vi "timeTest.vi"() -> ()   [LabVIEW 2019]
panel:
  out "czas":u32
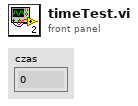
[diagram p1: front panel]
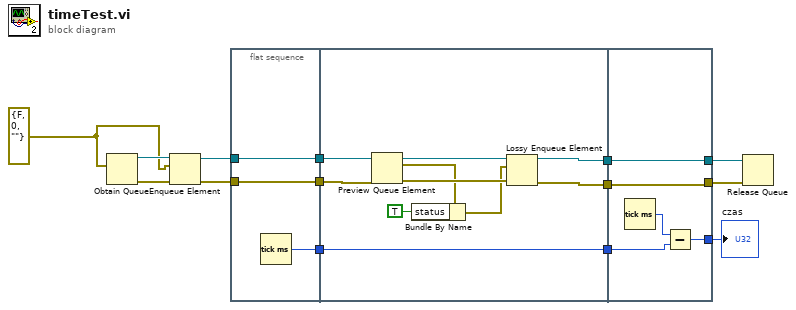
[diagram p0: block diagram]
diagram:
  w1 = errorcluster {"status"=FALSE, "code"=0, "source"=""} ("error constant")
  n1 = Obtain Queue(element data type=w1) -> (queue out=w14:refnum<queue>, error out=w13:errorcluster)  [unwired: 4 in, 1 out]
  n2 = Enqueue Element(queue=w14, element=w1, error in (no error)=w13) -> (queue out=w12:refnum<queue>, error out=w11:errorcluster)  [unwired: 1 in, 1 out]
  n3 = flat-sequence {
    tunnel: w11 -> [w16]
    tunnel: w12 -> [w17]
    tunnel: [w17] -> w10
    tunnel: [w16] -> w9
    tunnel: [w15] -> w8
    tunnel: w10 -> [w25]
    tunnel: w9 -> [w26]
    tunnel: w8 -> [w27]
    tunnel: [w27] -> w7
    tunnel: [w24] -> w5
    tunnel: [w23] -> w4
    tunnel: w7 -> [w31]
    tunnel: [w30] -> w6
    tunnel: w5 -> [w28]
    tunnel: [w29] -> w3
    tunnel: w4 -> [w29]
    tunnel: [w28] -> w2
    frame #0 {
      n4 = Tick Count (ms)() -> (millisecond timer value=w15:u32)
    }
    frame #1 {
      n5 = Preview Queue Element(queue=w25, error in (no error)=w26) -> (queue out=w21:refnum<queue>, element=w20:errorcluster, error out=w22:errorcluster)  [unwired: 1 in, 1 out]
      n6 = Bundle By Name(cluster=w20, "status"=TRUE) -> (w18:errorcluster)
      n7 = Lossy Enqueue Element(queue=w21, element=w18, error in (no error)=w22) -> (queue out=w24:refnum<queue>, error out=w23:errorcluster)  [unwired: 2 out]
    }
    frame #2 {
      n8 = Tick Count (ms)() -> (millisecond timer value=w32:u32)
      n9 = Subtract(x=w32, y=w31) -> (x-y=w30:u32)
    }
  }
  n10 = Release Queue(queue=w2, error in (no error)=w3) -> ()  [unwired: 1 in, 3 out]
  "czas" <- w6
